vi "TIO Data Stream Flatten.vi"(1 "Data Out":T1(array[cluster])=[{"Name"="gmr", "Waveform"={"start"=0.0, "dt"=1.0, "Timeseries"=[[-1045203.625, 2103369.25, -524451.0625]]}}, {"Name"="accel", "Waveform"={"start"=0.0, "dt"=1.0, "Timeseries"=[[0.4673272967338562, -9.214466094970703, -3.09728741645813]]}}, {"Name"="gyro", "Waveform"={"start"=0.0, "dt"=1.0, "Timeseries"=[[0.019417261704802513, 0.00881516095250845, 0.006293708924204111]]}}, {"Name"="bar", "Waveform"={"start"=0.0, "dt"=1.0, "Timeseries"=[[0.0]]}}, {"Name"="therm", "Waveform"={"start"=0.0, "dt"=1.0, "Timeseries"=[[0.0]]}}]) -> (0 "Flattened Array":dbl[][](array[numeric]))   [LabVIEW 2023]
panel:
  # "TIO Data Stream Flatten to Array"
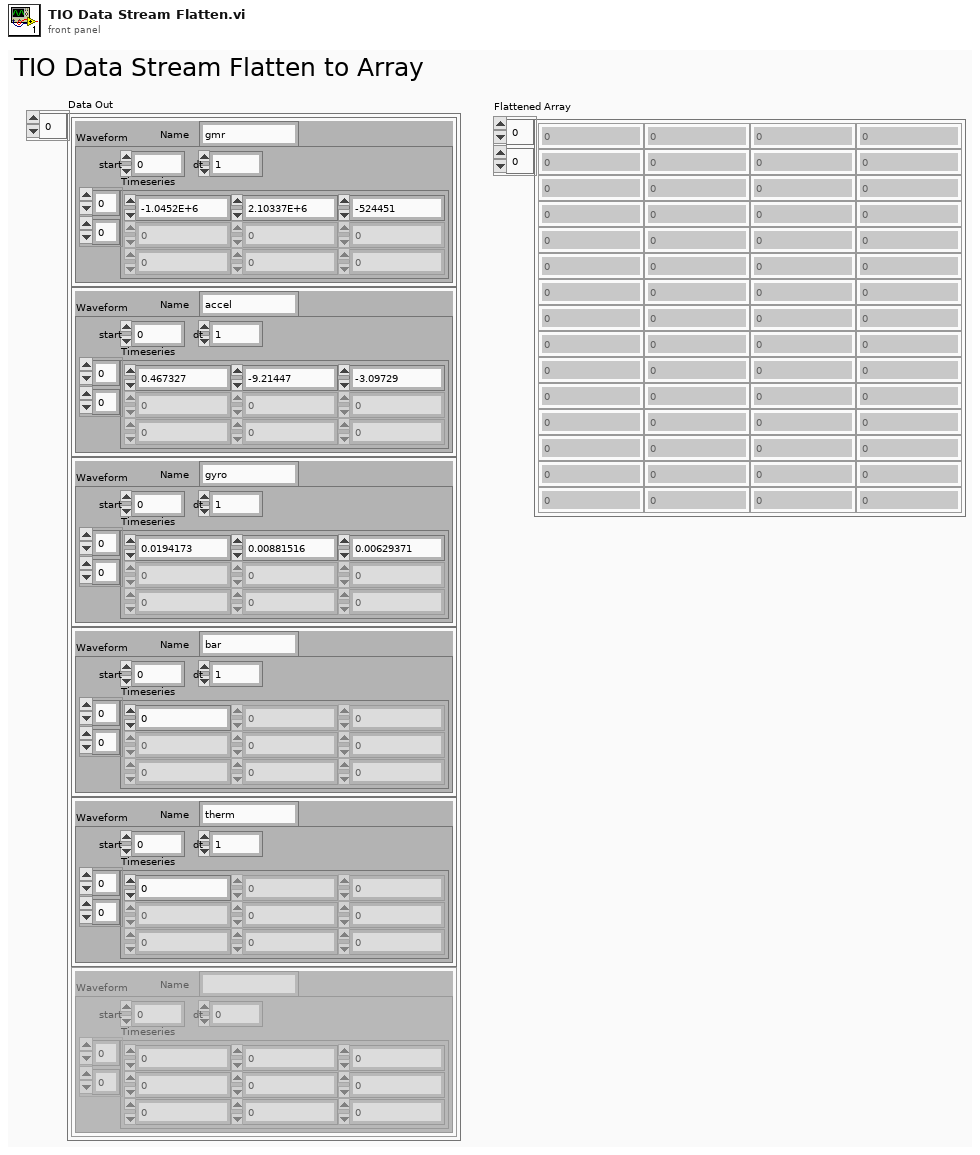
[diagram p1: front panel]
types:
  T1 = cluster{"Name":string, "Waveform":cluster{"start":dbl, "dt":dbl, "Timeseries":dbl[][]}}[]
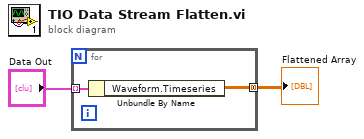
[diagram p0: block diagram]
diagram:
  n1 = for {
    tunnel: "Data Out" -> [w4] mode=indexing
    tunnel: [w3] -> w1 mode=concatenating
    n2 = Unbundle By Name(w4) -> ("Waveform.Timeseries"=w3:dbl[][])
  }
  "Flattened Array" <- w1
